vi "Downhill Simplex.vi"(5 "function data":T2, 7 "objective function":T3, 8 "error in (no error)":errorcluster, 9 "stopping criteria":T1={"function tolerance"=1e-06, "parameter tolerance"=1e-06, "max iterations"=100, "max function calls"=1000, "gradient tolerance"=1e-06, "max time (sec)"=-1.0}, 11 "start":dbl[](array[numeric])) -> (0 "error out":errorcluster, 1 "number of function evaluations":i32, 2 "f(minimum)":dbl, 3 "minimum":dbl[](array[numeric]))   [LabVIEW 2020, in "NI_Gmath.lvlib"]
doc: "Solves the unconstrained minimization problem for an arbitrary nonlinear function. You must manually select the polymorphic instance to use."
uses:
  <vilib>/gmath/NI_Gmath.lvlib
  <vilib>/gmath/NumericalOptimization/ucno_user objective function ref.ctl
  <vilib>/gmath/NumericalOptimization/objective function data.ctl
  <vilib>/gmath/NumericalOptimization/stopping criteria.ctl
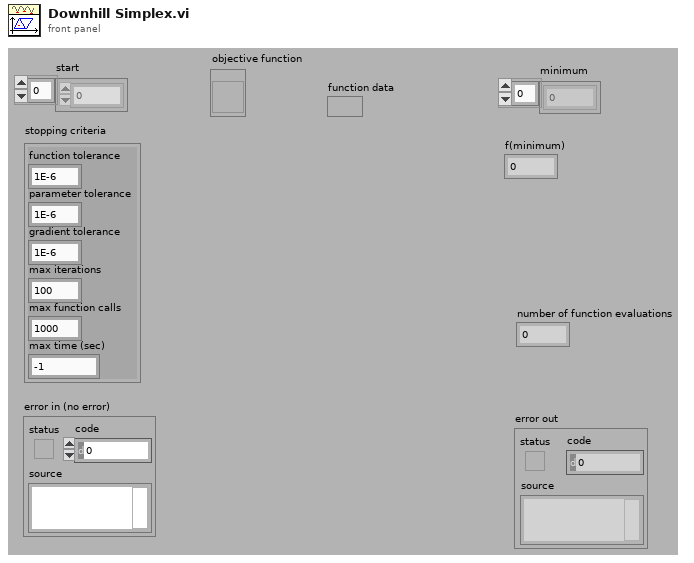
[diagram p1: front panel]
types:
  T1 = typedef "NI_Gmath.lvlib/stopping criteria.ctl" = cluster{"function tolerance":dbl, "parameter tolerance":dbl, "max iterations":i32, "max function calls":i32, "gradient tolerance":dbl, "max time (sec)":dbl}
  T2 = typedef "NI_Gmath.lvlib/objective function data.ctl" = variant
  T3 = typedef "NI_Gmath.lvlib/ucno_user objective function ref.ctl" = refnum<vi>
  T4 = typedef "NI_Gmath.lvlib/stopping criteria with time.ctl" = cluster{"function tolerance":dbl, "parameter tolerance":dbl, "max iterations":i32, "max function calls":i32, "gradient tolerance":dbl, "max time (sec)":dbl, "initial tick count":u32}
  T5 = cluster{"objective function":T3, "function data":T2}
  T6 = cluster{"objective function":bool, "gradient":bool}
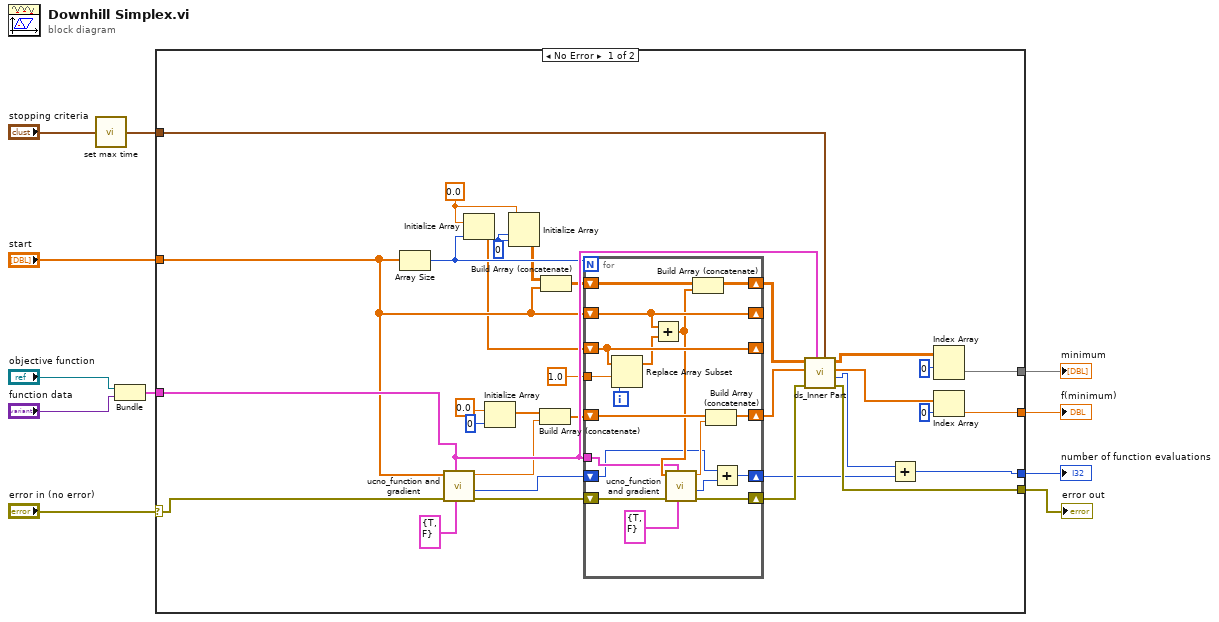
[diagram p0: block diagram]
diagram:
  n1 = call <vilib>:"set max time.vi"("stopping criteria"="stopping criteria") -> ("stopping criteria"=w1:T4)
  n2 = Bundle("objective function"="objective function", "function data"="function data") -> (w3:T5)  [unwired: 1 in]
  n3 = case shown="No Error" "error in (no error)" {
    selector: "error in (no error)" -> [w18 w62]
    tunnel: "start" -> [w42 _]
    tunnel: [w39 _] -> w10
    tunnel: [w36 _] -> w9
    tunnel: [w16 w62] -> w7
    tunnel: [w12 _] -> w6
    tunnel: w1 -> [w35 _]
    tunnel: w3 -> [w43 _]
    frame No Error {
      w24 = 0.0
      w28 = 0
      n4 = Array Size(array=w42) -> (size(s)=w27:i32)
      n5 = call <vilib>:"ucno_function and gradient.vi"("output control"=T6 {"objective function"=TRUE, "gradient"=FALSE}, "function and data"=w43, "error in (no error)"=w18, "X"=w42) -> ("error out"=w19:errorcluster, "number of function calls"=w17:i32, "f(X)"=w32:dbl)  [unwired: 4 in, 1 out]
      n6 = Initialize Array(w24, w27) -> (w23:dbl[])
      n7 = Initialize Array(0.0, 0) -> (w31:dbl[])
      n8 = Initialize Array(w24, w28, w28) -> (w25:dbl[][])
      n9 = Build Array (concatenate)(w31, w32) -> (w33:dbl[])
      n10 = Build Array (concatenate)(w25, w42) -> (w26:dbl[][])
      n11 = for {
        N: w27 -> [_]
        shift-right: [w60] -> w21
        shift-left: w26 -> [w61]
        shift-right: [w55] -> _
        shift-left: w42 -> [w55]
        shift-right: [w59] -> _
        shift-left: w23 -> [w59]
        tunnel: 1.0 -> [w51]
        shift-right: [w57] -> w22
        shift-left: w33 -> [w58]
        tunnel: w43 -> [w48]
        shift-right: [w50] -> w34
        shift-left: w19 -> [w49]
        shift-right: [w44] -> w13
        shift-left: w17 -> [w45]
        i -> [w52]
        n12 = Replace Array Subset(array=w59, new element=w51, index=w52) -> (w54:dbl[])
        n13 = Add(x=w55, y=w54) -> (x+y=w53:dbl[])
        n14 = call <vilib>:"ucno_function and gradient.vi"("output control"=T6 {"objective function"=TRUE, "gradient"=FALSE}, "function and data"=w48, "error in (no error)"=w49, "X"=w53) -> ("error out"=w50:errorcluster, "number of function calls"=w46:i32, "f(X)"=w56:dbl)  [unwired: 4 in, 1 out]
        n15 = Build Array (concatenate)(w61, w53) -> (w60:dbl[][])
        n16 = Build Array (concatenate)(w58, w56) -> (w57:dbl[])
        n17 = Add(x=w45, y=w46) -> (x+y=w44:i32)
      }
      n18 = call <vilib>:"ds_Inner Part.vi"("stopping criteria"=w35, "function and data"=w43, "error in"=w34, "f(Minimum) before"=w22, "Minimum before"=w21) -> ("error out"=w16:errorcluster, "number of function evaluations"=w14:i32, "f(Minimum) after"=w38:dbl[], "Minimum after"=w40:dbl[][])  [unwired: 2 in, 1 out]
      n19 = Add(x=w14, y=w13) -> (x+y=w12:i32)
      n20 = Index Array(array=w40, index (row)=0) -> (element=w39:dbl[])  [unwired: 1 in]
      n21 = Index Array(array=w38, index=0) -> (element=w36:dbl)
    }
    frame Error {
    }
  }
  "minimum" <- w10
  "f(minimum)" <- w9
  "error out" <- w7
  "number of function evaluations" <- w6
